vi "Simulation Call Statechart (VI).vi"(4 "operation":T14, 5 "Robot Index":i32, 8 "error in":errorcluster, 10 "Array of Sensors In":T1[](array[typedef]) {"Kobuki Sensors"."Infrared" format="%02x"; "iRobot Sensors"."Infrared" format="%02x"; "accelerometer"."z axis (g)" format="%.3f"; "accelerometer"."y axis (g)" format="%.3f"; "accelerometer"."x axis (g)" format="%.3f"}, 11 "simulator":T15={"configuration"={"maxTime"=5.0, "enableVisualization"=TRUE, "Environment Definition"=path "iRobot Navigation State Machine.vi", "Record Location"=path "Simulation Record.xml", "autograde?"=TRUE, "interactive?"=FALSE, "Feedback Mode"=enum."debug navigation", "Robot State Charts"=[path "C:/Users/blueuser/Desktop/Robo Sim Berkley/cpsgrader-release-0.4/Simulators/EECS149lab/src/LabVIEW/statechart/Simulation Statechart.vi"], "statechart"=path "C:/Users/blueuser/Desktop/Robo Sim Berkley/cpsgrader-release-0.4/Simulators/EECS149lab/src/LabVIEW/statechart/Simulation Statechart.vi"}, "Statechart\ndisplay"=refnum, "first step?"=FALSE, "Robots Simulation Statecharts"=[], "Robots"=[]}) -> (0 "error out":errorcluster, 2 "Array of Sensors Out":T1[](array[typedef]) {"Kobuki Sensors"."Infrared" format="%02x"; "iRobot Sensors"."Infrared" format="%02x"; "accelerometer"."z axis (g)" format="%.3f"; "accelerometer"."y axis (g)" format="%.3f"; "accelerometer"."x axis (g)" format="%.3f"}, 3 "simulator":T15={"configuration"={"maxTime"=5.0, "enableVisualization"=TRUE, "Environment Definition"=path "iRobot Navigation State Machine.vi", "Record Location"=path "Simulation Record.xml", "autograde?"=TRUE, "interactive?"=FALSE, "Feedback Mode"=enum."debug navigation", "Robot State Charts"=[path "C:/Users/blueuser/Desktop/Robo Sim Berkley/cpsgrader-release-0.4/Simulators/EECS149lab/src/LabVIEW/statechart/Simulation Statechart.vi"], "statechart"=path "C:/Users/blueuser/Desktop/Robo Sim Berkley/cpsgrader-release-0.4/Simulators/EECS149lab/src/LabVIEW/statechart/Simulation Statechart.vi"}, "Statechart\ndisplay"=refnum, "first step?"=FALSE, "Robots Simulation Statecharts"=[], "Robots"=[]})   [LabVIEW 2014]
uses:
  Simulator.ctl
  CyberSim interface/Simulation Configuration.ctl
  autograder/feedbackMode.ctl
  Multi Bot Code/RobotData.ctl
  <instrlib>/DC Motor Controller/HAIOL/DC Motor Controller.lvclass
  Simulation Call Statechart Operation.ctl
  shared/Sensors.ctl
  iRobot/Sensor/Accelerometer.ctl
  iRobot/Sensor/Sensor Group 6.ctl
  iRobot/Sensor/Bumps + Wheel Drops.ctl
  iRobot/Sensor/Buttons.ctl
  iRobot/Sensor/Charging State.ctl
  iRobot/Sensor/Charging Sources Available.ctl
  iRobot/Sensor/OI Mode.ctl
  iRobot/Sensor/Cargo Bay Digital Inputs.ctl
  iRobot/Sensor/Low-Side Driver + Wheel Overcurrent.ctl
  Kobuki/KobukiSensors.ctl
  Kobuki/Kobuki Bumps and WheelDrops.ctl
  Kobuki/Kobuki Buttons.ctl
  <vilib>/Statechart/Common/InstanceName.ctl
  <vilib>/Statechart/Common/DbgID.ctl
  <vilib>/Statechart/Common/IntGuid.ctl
  <vilib>/Statechart/Common/NI_SC_LVSCCommonFiles.lvlib
panel:
  # "Electrical: charging, battery, OI mode"
  # "Sensors: bump, cliff, button, wheel drop, wall, virtual wall"
  # "Motors:"
  # "Cargo Bay: I/O, overcurrent, infrared"
  # "Song"
  # "Inertia"
  # "Electrical: charging, battery, OI mode"
  # "Sensors: bump, cliff, button, wheel drop, wall, virtual wall"
  # "Motion: distance, angle, requested velocity"
  # "Cargo Bay: I/O, overcurrent, infrared"
  # "Song"
  # "Electrical: charging, battery, OI mode"
  # "Sensors: bump, cliff, button, wheel drop, wall, virtual wall"
  # "Motors:"
  # "Cargo Bay: I/O, overcurrent, infrared"
  # "Song"
  # "Inertia"
  # "Electrical: charging, battery, OI mode"
  # "Sensors: bump, cliff, button, wheel drop, wall, virtual wall"
  # "Motion: distance, angle, requested velocity"
  # "Cargo Bay: I/O, overcurrent, infrared"
  # "Song"
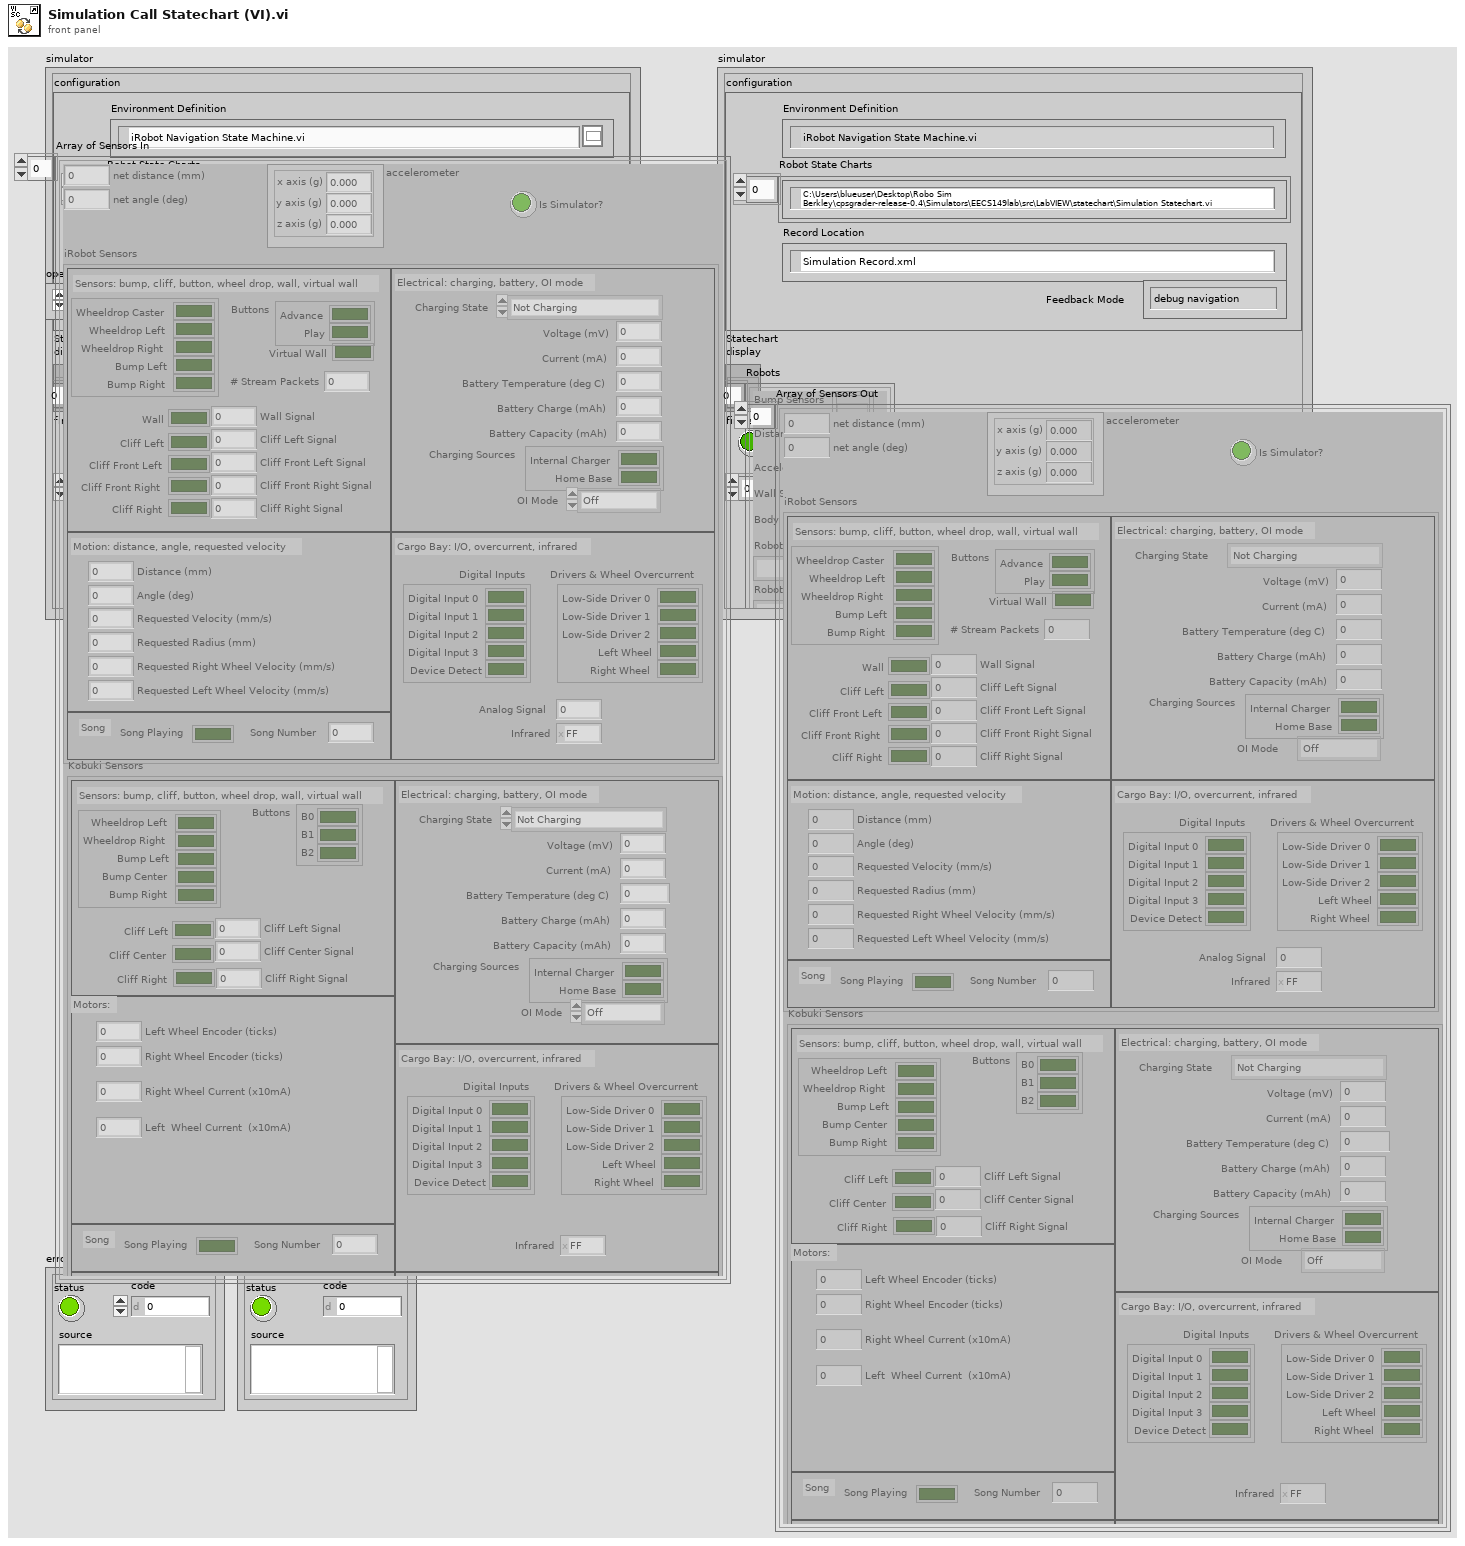
[diagram p1: front panel]
types:
  T1 = typedef "Sensors.ctl" = cluster{"net distance (mm)":i32, "net angle (deg)":i32, "accelerometer":T2, "iRobot Sensors":T3, "Is Simulator?":bool, "Kobuki Sensors":T11}
  T2 = typedef "Accelerometer.ctl" = cluster{"x axis (g)":dbl, "y axis (g)":dbl, "z axis (g)":dbl}
  T3 = typedef "Sensor Group 6.ctl" = cluster{"Bumps + Wheel Drops":T4, "Wall":bool, "Cliff Left":bool, "Cliff Front Left":bool, "Cliff Front Right":bool, "Cliff Right":bool, "Wall Signal":u16, "Cliff Left Signal":u16, "Cliff Front Left Signal":u16, "Cliff Front Right Signal":u16, "Cliff Right Signal":u16, "Buttons":T5, "Virtual Wall":bool, "# Stream Packets":u8, "Requested Velocity (mm/s)":i16, "Requested Radius (mm)":i16, "Requested Right Wheel Velocity (mm/s)":i16, "Requested Left Wheel Velocity (mm/s)":i16, "Distance (mm)":i32, "Angle (deg)":i32, "Song Playing":bool, "Song Number":u8, "Charging State":T6, "Voltage (mV)":u16, "Current (mA)":i16, "Battery Temperature (deg C)":i8, "Battery Charge (mAh)":u16, "Battery Capacity (mAh)":u16, "Charging Sources":T7, "OI Mode":T8, "Digital Inputs":T9, "Drivers & Wheel Overcurrent":T10, "Analog Signal":u16, "Infrared":u8}
  T4 = typedef "Bumps + Wheel Drops.ctl" = cluster{"Wheeldrop Caster":bool, "Wheeldrop Left":bool, "Wheeldrop Right":bool, "Bump Left":bool, "Bump Right":bool}
  T5 = typedef "Buttons.ctl" = cluster{"Advance":bool, "Play":bool}
  T6 = typedef "Charging State.ctl" = enum16{"Not Charging", "Reconditioning Charging", "Full Charging", "Trickle Charging", "Waiting", "Charging Fault Condition"}
  T7 = typedef "Charging Sources Available.ctl" = cluster{"Internal Charger":bool, "Home Base":bool}
  T8 = typedef "OI Mode.ctl" = enum16{"Off", "Passive", "Safe", "Full"}
  T9 = typedef "Cargo Bay Digital Inputs.ctl" = cluster{"Digital Input 0":bool, "Digital Input 1":bool, "Digital Input 2":bool, "Digital Input 3":bool, "Device Detect":bool}
  T10 = typedef "Low-Side Driver + Wheel Overcurrent.ctl" = cluster{"Low-Side Driver 0":bool, "Low-Side Driver 1":bool, "Low-Side Driver 2":bool, "Left Wheel":bool, "Right Wheel":bool}
  T11 = typedef "KobukiSensors.ctl" = cluster{"Bumps + Wheel Drops":T12, "Cliff Left":bool, "Cliff Center":bool, "Cliff Right":bool, "Cliff Left Signal":i16, "Cliff Center Signal":i16, "Cliff Right Signal":i16, "Buttons":T13, "Left Wheel Encoder (ticks)":i16, "Song Playing":bool, "Song Number":u8, "Charging State":T6, "Voltage (mV)":i16, "Current (mA)":i16, "Battery Temperature (deg C)":i16, "Battery Charge (mAh)":i16, "Battery Capacity (mAh)":i16, "Charging Sources":T7, "OI Mode":T8, "Digital Inputs":T9, "Drivers & Wheel Overcurrent":T10, "Infrared":u8, "Right Wheel Encoder (ticks) ":i16, "TimeStamp":u16, "Right Wheel Current (x10mA)":i16, "Left  Wheel Current  (x10mA)":i16, "Angle( of 100deg)":i16, "Angle Rate( of 100 deg/sec)":i16}
  T12 = typedef "Kobuki Bumps and WheelDrops.ctl" = cluster{"Wheeldrop Left":bool, "Wheeldrop Right":bool, "Bump Left":bool, "Bump Center":bool, "Bump Right":bool}
  T13 = typedef "Kobuki Buttons.ctl" = cluster{"B0":bool, "B1":bool, "B2":bool}
  T14 = typedef "Simulation Call Statechart Operation.ctl" = enum16{"Initialize", "Call Statechart", "Finalize"}
  T15 = typedef "Simulator.ctl" = cluster{"configuration":T16, "Statechart\ndisplay":refnum<vi>, "first step?":bool, "Robots Simulation Statecharts":path[], "Robots":T18[]}
  T16 = typedef "Simulation Configuration.ctl" = cluster{"maxTime":sgl, "enableVisualization":bool, "Environment Definition":path, "Record Location":path, "autograde?":bool, "interactive?":bool, "Feedback Mode":T17, "Robot State Charts":path[], "statechart":path}
  T17 = typedef "feedbackMode.ctl" = enum32{"debug navigation", "debug hill climb", "autograde navigation", "autograde hill climb"}
  T18 = typedef "RobotData.ctl" = cluster{"Bump Sensors":refnum<k20>[], "Distance Sensors":refnum<k20>[], "Accelerometer":refnum<k20>, "Wall Sensor":refnum<k20>, "Body":refnum<k20>, "RobotID":string, "RobotType":string, "Left Motor":refnum<class "DC Motor Controller.lvclass">, "Right Motor":refnum<class "DC Motor Controller.lvclass">}
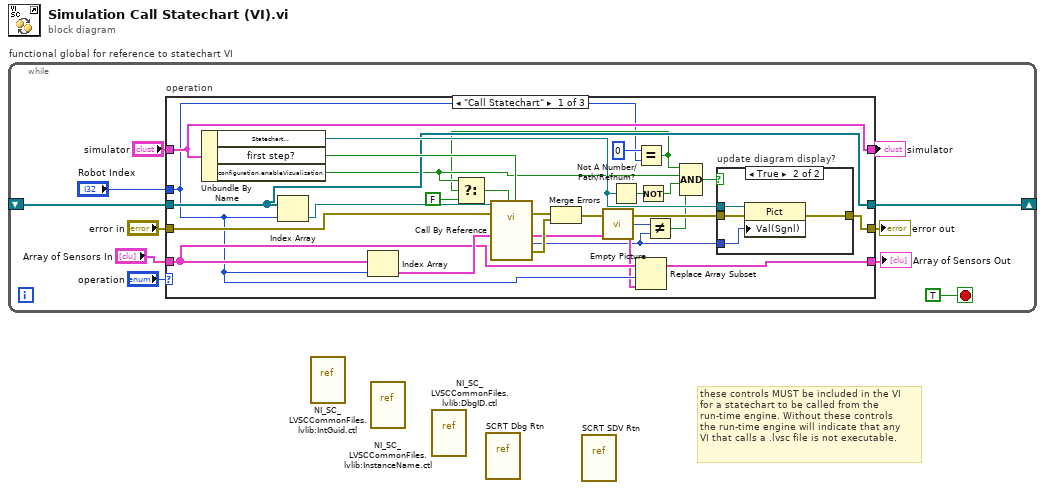
[diagram p0: block diagram]
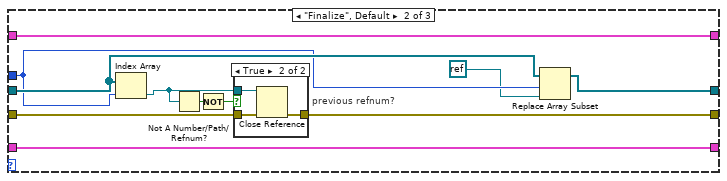
[diagram p3: hidden frame]
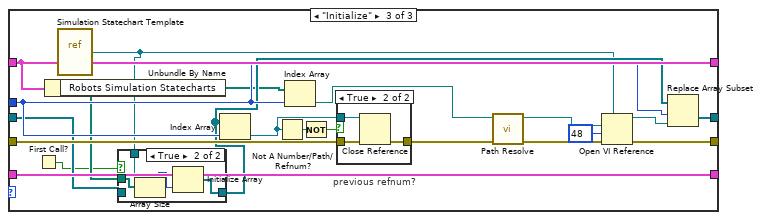
[diagram p5: hidden frame]
diagram:
  # "these controls MUST be included in the VI\nfor a statechart to be called from the\nrun-time engine. Without these controls\nthe run-time engine will indicate that any\nVI that calls a .lvsc file is not executable."
  n1 = while "functional global for reference to statechart VI" {
    shift-right: [w4] -> _
    shift-left: _ -> [w5]
    stop <- TRUE stop-if-true
    n2 = case "operation" shown="\"Call Statechart\"" "operation" {
      tunnel: [w32 w51 w77] -> w6
      tunnel: "error in" -> [w31 w52 w76]
      tunnel: "simulator" -> [w28 w53 w74]
      tunnel: [w18 w50 w75] -> w1
      tunnel: [w28 w53 w74] -> w7
      tunnel: "Array of Sensors In" -> [w17 w50 w75]
      tunnel: w5 -> [w25 w46 w62]
      tunnel: [w25 w43 w64] -> w4
      tunnel: "Robot Index" -> [w16 w45 w63]
      frame "Call Statechart" {
        n3 = Unbundle By Name(w28) -> ("Statechart\ndisplay"=w34:refnum<vi>, "first step?"=w27:bool, "configuration.enableVisualization"=w23:bool)
        n4 = Index Array(array=w25, index=w16) -> (element=w26:refnum<vi>)
        n5 = Index Array(array=w17, index=w16) -> (element=w19:T1)
        n6 = call "Empty Picture"() -> ("empty picture"=w12:picture)
        n7 = Not A Number/Path/Refnum?(number/path/refnum=w34) -> (NaN/Path/Refnum?=w36:bool)
        n8 = Equal?(x=0, y=w16) -> (x = y?=w22:bool)
        n9 = Select(t=w23, s=w22, f=FALSE) -> (s? t:f=w20:bool)
        n10 = call-by-ref "Call By Reference"(reference=w26, error in=w31, "firstStep?"=w27, "enableVisualization?"=w20, "sensors"=w19) -> (error out=w30:errorcluster, 0:"error out"=w29:errorcluster, "Diagram Display"=w14:picture, "sensors"=w15:T1)  [unwired: 6 in, 1 out]
        n11 = Merge Errors(w30, w29) -> (w33:errorcluster)
        n12 = Replace Array Subset(array=w17, new element=w15, index=w16) -> (w18:T1[])
        n13 = Not(x=w36) -> (.not. x?=w37:bool)
        n14 = Not Equal?(x=w12, y=w14) -> (x != y?=w13:bool)
        n15 = Compound Arithmetic op=AND(w22, w23, w37, w13) -> (w35:bool)
        n16 = case "update diagram display?" shown="True" w35 {
          tunnel: w34 -> [_ w42]
          tunnel: w33 -> [w38 w41]
          tunnel: [w38 w40] -> w32
          tunnel: w14 -> [_ w39]
          frame False {
          }
          frame True {
            n17 = property class="Pict"(reference=w42, error in=w41, "Val(Sgnl)"=w39) -> (error out=w40:errorcluster)  [unwired: 1 out]
          }
        }
      }
      frame "Finalize", Default {
        n18 = Index Array(array=w46, index=w45) -> (element=w47:refnum<vi>)
        n19 = Not A Number/Path/Refnum?(number/path/refnum=w47) -> (NaN/Path/Refnum?=w48:bool)
        n20 = Not(x=w48) -> (.not. x?=w49:bool)
        n21 = case "previous refnum?" shown="True" w49 {
          tunnel: w52 -> [w54 w57]
          tunnel: [w54 w56] -> w51
          tunnel: w47 -> [_ w55]
          frame False {
          }
          frame True {
            n22 = Close Reference(reference=w55, error in (no error)=w57) -> (error out=w56:errorcluster)
          }
        }
        n23 = Replace Array Subset(array=w46, new element=refnum<k0> refnum, index=w45) -> (w43:refnum<vi>[])
      }
      frame "Initialize" {
        n24 = First Call?() -> (First Call?: T/F=w58:bool)
        n25 = Unbundle By Name(w74) -> ("Robots Simulation Statecharts"=w59:path[])
        n26 = vi-ref "Simulation Statechart Template.vi"() -> (w60:refnum<vi>)
        n27 = case shown="True" w58 {
          tunnel: w62 -> [w78 _]
          tunnel: [w78 w79] -> w61
          tunnel: w60 -> [_ w82]
          tunnel: w59 -> [_ w80]
          frame False {
          }
          frame True {
            n28 = Array Size(array=w80) -> (size(s)=w81:i32)
            n29 = Initialize Array(w82, w81) -> (w79:refnum<vi>[])
          }
        }
        n30 = Index Array(array=w61, index=w63) -> (element=w67:refnum<vi>)
        n31 = Not A Number/Path/Refnum?(number/path/refnum=w67) -> (NaN/Path/Refnum?=w71:bool)
        n32 = Index Array(array=w59, index=w63) -> (element=w66:path)
        n33 = Not(x=w71) -> (.not. x?=w70:bool)
        n34 = case "previous refnum?" shown="True" w70 {
          tunnel: w76 -> [w83 w86]
          tunnel: [w83 w85] -> w69
          tunnel: w67 -> [_ w84]
          frame False {
          }
          frame True {
            n35 = Close Reference(reference=w84, error in (no error)=w86) -> (error out=w85:errorcluster)
          }
        }
        n36 = call "Path Resolve.vi"("Error In"=w69, "absolute or relative path"=w66) -> ("Error Out"=w73:errorcluster, "resolved path"=w72:path)  [unwired: 8 in]
        n37 = Open VI Reference(type specifier VI Refnum (for type only)=w60, vi path=w72, options=48, error in (no error)=w73) -> (vi reference=w65:refnum<vi>, error out=w77:errorcluster)  [unwired: 2 in]
        n38 = Replace Array Subset(array=w61, new element=w65, index=w63) -> (w64:refnum<vi>[])
      }
    }
    "simulator" <- w7
    "error out" <- w6
    "Array of Sensors Out" <- w1
  }
  n39 = vi-ref "NI_SC_LVSCCommonFiles.lvlib:IntGuid.ctl"() -> ()  [unwired: 1 out]
  n40 = vi-ref "NI_SC_LVSCCommonFiles.lvlib:InstanceName.ctl"() -> ()  [unwired: 1 out]
  n41 = vi-ref "NI_SC_LVSCCommonFiles.lvlib:DbgID.ctl"() -> ()  [unwired: 1 out]
  n42 = vi-ref <vilib>:"SCRT Dbg Rtn.vi"() -> ()  [unwired: 1 out]
  n43 = vi-ref <vilib>:"SCRT SDV Rtn.vi"() -> ()  [unwired: 1 out]
